vi "AlliGator Add Dataset to Accumulated Dataset.vi"(8 "error in (no error)":errorcluster, 9 "Weight (1)":dbl=1.0, 11 "AlliGator IV DVR in":refnum<data-value>) -> (0 "error out":errorcluster, 3 "AlliGator IV DVR out":refnum<data-value>)   [LabVIEW 2021, in "AlliGator Accumulated Dataset.lvlib"]
doc: "Adds the <B>Current Dataset</B> to the <B>Accumulated Dataset</B>, if and only if the number of gates and channels are the same as those of the first dataset in the series.\n\nIf not, the <B>Current Dataset</B> is skipped."
uses:
  AlliGator Accumulated Dataset.lvlib
  Internal Variables/AlliGator Internal Variables v2.ctl
  <vilib>/vision/Image Controls.llb/IMAQ Image.ctl
  Internal Variables/AlliGator Gate Image Set.ctl
  Files/AlliGator FLI Dataset Type.ctl
  Files/AlliGator Data Series Type.ctl
  Dual-Channel Datasets/AlliGator Dataset Channel.ctl
  Settings/AlliGator Gate Arithmetic.ctl
  Source Image/AlliGator Displayed Image.ctl
  Image/Named ROI Description.ctl
  Phasor Graph/AlliGator Decay Metadata v3.ctl
  Decay Analysis/Decay Preprocessing/AlliGator Decay Background Subtraction Info.ctl
  Decay Analysis/Decay Preprocessing/AlliGator Baseline Subtraction Method.ctl
  Graphs/XY Graph/XY Graph Plot Shift Parameters.ctl
  Graphs/XY Graph/XY Graph Plot Shift Method.ctl
  Decay Analysis/Decay Preprocessing/AlliGator Decay Extrapolation Parameters.ctl
  Phasor/Calibration Phasor (m, phi).ctl
  Phasor/Phasor Reference Series.ctl
  Phasor/Phasor Calibration Map v2.ctl
  Phasor/Phasor (g, s).ctl
  Phasor Graph/AlliGator Raw Phasor Plot Data v5.ctl
  Phasor/Phasor Standard Deviation Options.ctl
  Phasor Plot/AlliGator Phasor Multi-Harmonic Data.ctl
  Phasor/Phasor Harmonic Data.ctl
  Decay Fit Parameter Map/AlliGator Decay Fit Options & Parameters v4.ctl
  Fits/IRF(X)PSED/Decay Fit Options v4.ctl
  Fits/Decay Convolution/Decay Model.ctl
  Fits/Residual Type.ctl
  Fits/IRF(X)PSED/Fit Weights Type v2.ctl
  Fits/Non-linear Fitting Method v2.ctl
  Fits/Fit Calculation Method.ctl
  Fits/Non-linear Fitting Algorithm.ctl
  Decay Analysis/Decay Fit/AlliGator Decay Fit Parameter Constraints 2.ctl
  Fits/IRF(X)PSED/Decay Fit Parameters In List.ctl
  Fits/IRF(X)PSED/MLE Baseline Offset Type.ctl
  Decay Analysis/Decay Preprocessing/AlliGator Decay Preprocessing Parameters.ctl
  Fits/IRF(X)PSED/Decay Fit Parameters & Derived Quantities List v2.ctl
  Fits/IRF(X)PSED/Decay Fit Result Constraint.ctl
  Decay Fit Parameter Map/AlliGator Parameter Maps Data.ctl
  Globals, Variables, Constants/AlliGator Variables List.ctl
  Rich Text Box/Text Format List.ctl
  <vilib>/vision/NI_Vision_Development_Module.lvlib
  Globals, Variables, Constants/AlliGator Globals, Variables & Constants.lvlib
  Notebook/Notebook.lvlib
  Utilities/Utilities.lvlib
  Image/Image.lvlib
  Phasor/Phasor.lvlib
  Internal Variables/AlliGator Internal Variables.lvlib
  Files/AlliGator Files.lvlib
  Phasor Graph/AlliGator Phasor Graph.lvlib
  Decay Analysis/Decay Preprocessing/AlliGator Decay Preprocessing.lvlib
  Graphs/XY Graph/XY Graph Add-Ons.lvlib
  Phasor Plot/AlliGator Phasor Plot.lvlib
  Source Image/AlliGator Source Image.lvlib
  Fits/Fits.lvlib
  Decay Analysis/Decay Fit/AlliGator Decay Fit.lvlib
  Settings/AlliGator Settings.lvlib
  Dual-Channel Datasets/AlliGator Dual-Channel Datasets.lvlib
  Decay Fit Parameter Map/AlliGator Decay Fit Parameter Map.lvlib
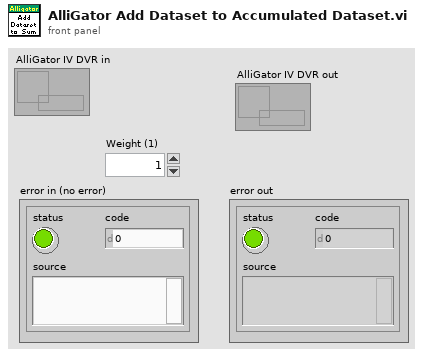
[diagram p1: front panel]
types:
  T1 = typedef "AlliGator Globals, Variables & Constants.lvlib/AlliGator Variables List.ctl" = enum16{"---- GUI ----", "GUI:Initialization Status", "GUI:State Indicators Refnum", "GUI:Original AlliGator Menu Items", "GUI:Current Action Loop State", "GUI:Script in progress", "GUI:Playback", "GUI:Loop Playback", "GUI:Search ROI Used", "GUI:Search ROI", "Decay Graph Max Legend Size", "Intensity Graph Max Legend Size", "Decay Statistics Graph Max Legend Size", "Phasor Graph Max Legend Size", "Phasor Ratio Graph Max Legend Size", "Lifetime Graph Max Legend Size", "---- Files ----", "Files:Export Dataset Frames as Individual Files", "Files:Show Batch Export Help Balloons", "Files:Frames in Dataset", "Files:ptu File Frame Start Indices", "Files:Current Frame in Dataset", "Files:Current Frame Timestamp", "Files:Dataset Loaded", "Files:Dataset Metadata", "Files:Dataset Channel", "Files:Dataset Data Description", "Files:Background Dataset Metadata", "Files:Background Dataset Channel", "Files:Background Dataset Data Description", "Files:Background File Subtraction", "Files:Background File Path", "Files:Background File Pile-up Correction", "Files:Background File Pixel Well Capacity", "Files:Background File Scaling Factor", "Files:Current Dataset Load Settings", "Files:Dataset Path", "Files:ICCD-specific Information", "Files:Macrotime Gate Separation", "------ Python Plugins ------", "Python Plugins:Information", "Python Plugins:Python Session", "Python Plugins:Valid Python Session?", "---- Source Image ----", "Source Image:ROIs", "Source Image:Current ROI", "Source Image:ROI Event Refnum", "X_Source Image:Display Range", "X_Source Image:Palette Information", "X_Source Image:Type of Displayed Image", "X_Time Gate Slider", "Source Image:Palette List", "Source Image:Scale", "Source Image:ROI Overlay Color", "Source Image:Overlay to Erase", "Source Image:Is Displayed Image Accumulated", "Source Image:White Light Image Modified", "Source Image:Mask Image Modified", "---- Image Profile Window ----", "Image Profile:Window Event Refnum", "Image Profile:IntensityType", "Image Profile:Intensity Average Type", "Image Profile:Intensity-weighted SDV", "Image Profile:Box Profile Type", "Image Profile:Window Open", "Image Profile:Plotted Fit Parameter", "------ Phasor Graph -------", "Phasor Graph:Show Line", "---- Phasor Plot ---", "Phasor Plot:Parameters Changed", "Phasor Plot:FLI Dataset Modified since last Calculation", "Phasor Harmonics Data", "Selected Phasor Harmonics", "Phasor Harmonic Manager Event Refnum", "Phasor Plot:ROIs", "Phasor Plot:Current ROI", "Phasor Plot:ROI Event Refnum", "Phasor Plot:Image Reference Points", "Phasor Plot:Computed", "Phasor Plot:Palette Information", "Phasor Plot:Palette List", "Phasor Plot:Phasor Ratio Palette Information", "Phasor Plot:Phasor Ratio Palette List", "Phasor Plot:Image Scale", "Phasor Plot:Image Overlay to Erase", "Phasor Plot:Image Elements to Update", "Phasor Plot:Current Calculation Parameters", "Phasor Plot:Current Calibration Options", "Phasor Plot:Reset Cumulated Phasor Plot", "Phasor Plot:Reference 1", "Phasor Plot:Lifetime Reference 1", "Phasor Plot:Reference 1 Frequency", "Phasor Plot:Reference 2", "Phasor Plot:Lifetime Reference 2", "Phasor Plot:Reference 2 Frequency", "---- Decay Analysis ----", "Number of Selected Decays to Fit", "LS Fit Results", "LAR Fit Results", "BS Fit Results", "Last Decay Max - Min", "Best Fit Parameters", "Best Fit Parameter Names", "Actual Size X", "Actual Size Y", "Binning X", "Binning Y", "Actual # Gates", "Dataset Number", "Gates to...", "Gates Skipped", "Gates to keep", "Gate Step", "Gate Separation", "Reversed Gates", "Pile-up Correction", "Pixel Well Capacity", "Background Subtracted", "Background Subtraction Method", "Background Definition Range", "Background File (deprecated)", "Number of Dataset Accumulated", "Array of Accumulated Dataset Paths", "Do Averaged Datasets", "Destination File Path", "Process Plot Target", "Use 1/D as Phasor Frequency", "---- Decay Fit Parameter Map -----", "Decay Fit Parameter Map:Palette Information", "Decay Fit Parameter Map:Palette List", "Decay Fit Parameter Map:X Resolution", "Decay Fit Parameter Map:Y Resolution", "Decay Fit Parameter Map:Use Decay Fit Result Constraints", "Decay Fit Parameter Map:Decay Fit Result Constraints", "Decay Fit Parameter Map:Decay Fit Result Constraints Applied", "---- Parameter Map ----", "Parameter Map:Palette Information", "Parameter Map:Palette List", "------- Local Decay Window ---------", "Local Decay Graph Window:Event Refnum", "Local Decay Graph Window:Use normalized IRF for convolution", "----- Miscellaneous ----", "Misc:Skippable Dialog Windows Status"}
  T2 = enum32{"Average", "Min", "Max", "Clear  if < ", "Clear  if < or =", "Clear  if =", "Clear  if > or =", "Clear  if >"}
  T3 = typedef "Notebook.lvlib/Text Format List.ctl" = enum16{"Message", "Result", "Error", "Setting", "Verbose", "Warning"}
  T4 = typedef "AlliGator Internal Variables.lvlib/AlliGator Internal Variables v2.ctl" = cluster{"----------------------------- Images -----------------------------":u8, "Displayed Image":T5, "White Light Image":T5, "Mask Image":T5, "ROI Mask Image":T5, "Current Dataset Images 1":T6, "Background Dataset Images 1":T6, "Current Dataset Images 2":T6, "Background Dataset Images 2":T6, "Current Dataset Arithmetic Images":T6, "Accumulated Dataset Images 1":T6, "Accumulated Dataset Images 2":T6, "Accumulated Dataset Arithmetic Images":T6, "----------------------------- File Paths -----------------------------":u8, "Phasor Plot Image":T5, "Decay Fit Parameter Map Image":T5, "Parameter Map Image":T5, "Single Data Point Path":path, "White Light Image Path":path, "Mask Image Path":path, "Time-Series Folder":path, "[Time-Series Paths]":path[], "----------------------------- FLI Dataset -----------------------------":u8, "Current Dataset":i32, "Single Dataset Type":T7, "Current Folder":string, "AlliGator Data Series Type":T8, "# Datasets":i32, "Dual-Channel Dataset":bool, "Selected Channel Name":string, "Dataset Channel":T9, "Channel Arithmetic":T10, "Dual-Channel Background Dataset":bool, "Background Channel":T9, "Dual-Channel Accumulated Dataset":bool, "Start Time":dbl, "[Time-Series Timestamps]":dbl[], "[Intensity Corrections]":dbl[], "Time Series Script":bool, "Type of Displayed Image":T11, "Gate Image Slide":u16, "# Gates":i32, "ROIs":T12[], "----------------------------- Decays -----------------------------":u8, "ROI Decay":cluster{"t Array":dbl[], "I Array":dbl[]}, "Valid Decay":bool, "Decay  Metadata":T14, "Reference Decay Plot Name":string, "Reference Decay":cluster{"t Array":dbl[], "I Array":dbl[]}, "Decay Shift Plot":cluster{"Time Stamps":dbl[], "Decay Shifts":dbl[]}, "[Decays Max Values]":sgl[], "[Decays Min Values]":sgl[], "----------------------------- Calibration -----------------------------":u8, "Calibration Phasor":T20, "Calibration Phasor Series":T21, "Phasor Calibration Map":T22, "Calibration Map MD5 Digest":string, "----------------------------- Phasor Graph -----------------------------":u8, "Last Raw Phasor":T23, "Last Calibrated Phasor":T23, "Last Calibrated Phasor SDV":T23, "Phasor Graph:Phasor Plot":cluster{"g Array":dbl[], "s Array":dbl[]}, "Phasor Graph:Phasor SDV Plot":cluster{"g Array":dbl[], "s Array":dbl[]}, "[Phasor Graph:Raw Phasor Plots]":T24[], "Phasor Plot locked to Ref 1":i32, "[Phasor Plot(s) locked to Ref 1]":i32[], "[Phasor Plot(s) locked to Ref 2]":i32[], "[Pixel Phasors]":T23[], "----------------------------- Phasor Plot -----------------------------":u8, "[[Sum Image]]":dbl[][], "[[CSG Phasors]]":csg[][], "[[Valid Pixel?]]":bool[][], "[[Phasor Ratios]]":dbl[][], "[[Average Lifetimes]]":dbl[][], "Amplitude Weighted Average Lifetime":bool, "I/m/phi Dataset":cluster{"I/m/phi Dataset?":bool, "Base Frequency":dbl[unit], "Harmonic Orders":u8[]}, "Multi Phasor Plot Data":T26, "----------------------------- Decay Fit Parameter Map -----------------------------":u8, "Decay Fit Options & Parameters":T28, "Fit Options: Decay Preprocessing Parameters":T39, "Fit Options: Reference Decay":cluster{"t Array":dbl[], "I Array":dbl[]}, "Is Full Image Parameters Map":bool, "Is Single-Pixels Parameters Map":bool, "NLSF Parameters Map X Resolution":i32, "NLSF Parameters Map Y Resolution":i32, "[Single Decay Fit Parameters]":dbl[], "Fit Model":T30, "[[Multiple Decays Fit Parameters]]":dbl[][], "[[Multiple Decays Fit Parameter SDVs]]":dbl[][], "[[IRFs]]":dbl[][], "[ROI Descriptors]":T13[], "IRF Array Time Axis":dbl[], "Decay Array Time Axis":dbl[], "[Decay Fit Parameter Names]":T40[], "[Decay Sum]":dbl[], "Array of Decay Fit Result Constraints":T41[], "Selected ROIs Array":bool[], "----------------------------- Parameter Maps -----------------------------":u8, "[Map Set Names]":string[], "[Parameter Maps]":T42[], "[[User-defined Quantities]]":dbl[][], "User-defined Quantity":string}
  T5 = typedef "IMAQ Image.ctl" = refnum<image>
  T6 = typedef "AlliGator Internal Variables.lvlib/AlliGator Gate Image Set.ctl" = cluster{"SGL Gate Images":T5[], "SGL Sum Image":T5, "SGL Max Image":T5, "SGL Min Image":T5}
  T7 = typedef "AlliGator Files.lvlib/AlliGator FLI Dataset Type.ctl" = enum16{"HDF5 FLI Dataset", "Gate Image Folder", ".sdt FLI Dataset (Becker & Hickl)", ".ptu FLI Dataset (PicoQuant)", "SS1 FLI Dataset", "SS2 FLI Dataset", "I/m/phi Dataset", ".bin FLI Dataset (PicoQuant Binned)", ".bin FLI Dataset (Piccolo Binned)", ".mat FLI Dataset"}
  T8 = typedef "AlliGator Files.lvlib/AlliGator Data Series Type.ctl" = enum16{"Not a Supported Series", "Gate Images Folder Series", "SwissSPAD 2 Dataset Series", "B&H FLI Dataset Series", "PicoQuant PTU FLI Dataset Series", "PicoQuant BIN FLI Dataset Series", "Piccolo hist BIN FLI Dataset Series", "HDF5 FLI Dataset Series"}
  T9 = typedef "AlliGator Dual-Channel Datasets.lvlib/AlliGator Dataset Channel.ctl" = enum16{"G2", "INT"}
  T10 = typedef "AlliGator Settings.lvlib/AlliGator Gate Arithmetic.ctl" = enum16{"None", "INT-G2", "G2/INT*<INT>", "(1 - G2/INT)*<INT>"}
  T11 = typedef "AlliGator Source Image.lvlib/AlliGator Displayed Image.ctl" = enum16{"Single Gate", "Sum of All Gates", "Max of All Gates", "Min of All Gates", "-", "White Ligth Image", "Mask Image"}
  T12 = typedef "Image.lvlib/Named ROI Description.ctl" = cluster{"ROI Descriptor":T13, "ROI Name":string, "Overlay Color":u32}
  T13 = typedef "ROI Descriptor" = cluster{"Global Rectangle":i32[], "Contours":cluster{"ID":enum32{"External", "Internal"}, "Type":u32, "Coordinates":i32[]}[]}
  T14 = typedef "AlliGator Phasor Graph.lvlib/AlliGator Decay Metadata v3.ctl" = cluster{"ROI Descriptor":T13, "ROI Center":cluster{"X":i32, "Y":i32}, "Decay Background Subtraction Info":T15, "Decay Reverted":bool, "Decay Smoothened":bool, "Decay Straightened":bool, "Fitted Tau (Decay Straightening)":dbl, "Decay Shift Parameters":T17, "Decay Shifted":bool, "Decay Extrapolated":bool, "Decay Extrapolation Parameters":T19, "Decay Normalized":bool, "Fold Decay":bool, "# Folds":u32}
  T15 = typedef "AlliGator Decay Preprocessing.lvlib/AlliGator Decay Background Subtraction Info.ctl" = cluster{"Laser Period":dbl[unit], "Gate Duration":dbl[unit], "Baseline Subtraction Method":T16, "Background Definition Range":cluster{"Min Gate":dbl[unit], "Max Gate":dbl[unit]}, "Total Intensity w/o Bkgd Subtraction":dbl, "Bkgd-subtracted Intensity (exp)":dbl, "# Data Points":i32, "Background/Gate":dbl, "Fitted Lifetime":dbl[unit], "Bkgd-subtracted Intensity (theo)":dbl}
  T16 = typedef "AlliGator Decay Preprocessing.lvlib/AlliGator Baseline Subtraction Method.ctl" = enum16{"Mean", "Min", "Square Gated Single-Exponential", "File", "Constant"}
  T17 = typedef "XY Graph Add-Ons.lvlib/XY Graph Plot Shift Parameters.ctl" = cluster{"Type":T18, "Shift":dbl[unit], "Threshold":dbl, "Rotate":bool}
  T18 = typedef "XY Graph Add-Ons.lvlib/XY Graph Plot Shift Method.ctl" = enum16{"Default", "CFD", "Threshold", "Cross-Correlation"}
  T19 = typedef "AlliGator Decay Preprocessing.lvlib/AlliGator Decay Extrapolation Parameters.ctl" = cluster{"Additional Points":u32, "Head Fraction":dbl, "Fitted Tau":dbl, "Use Periodicity":bool, "Use Cursors":bool, "Tail Fraction":dbl}
  T20 = typedef "Phasor.lvlib/Calibration Phasor (m, phi).ctl" = cluster{"m":dbl, "phi":dbl, "Phasor Frequency":dbl[unit], "Reference Lifetime":dbl[unit]}
  T21 = typedef "Phasor.lvlib/Phasor Reference Series.ctl" = cluster{"m Array":dbl[], "phi Array":dbl[], "Phasor Frequency":dbl[unit], "Calibration Lifetime":dbl[unit]}
  T22 = typedef "Phasor.lvlib/Phasor Calibration Map v2.ctl" = cluster{"Phasor Frequency":dbl[unit], "Calibration Lifetime":dbl[unit], "ROI Centers":cluster{"X":i32, "Y":i32}[], "ROI Descriptors":T13[], "Map Resolution X":i32, "Map Resolution Y":i32, "z Array":cdb[]}
  T23 = typedef "Phasor.lvlib/Phasor (g, s).ctl" = cluster{"g":dbl, "s":dbl}
  T24 = typedef "AlliGator Phasor Graph.lvlib/AlliGator Raw Phasor Plot Data v5.ctl" = cluster{"Phasor Plot Name":string, "Raw Phasor Plot":T23[], "Phasor Frequency":dbl[unit], "[Decay Metadata]":T14[], "Raw Phasor Plot SDV":T23[], "Phasor SDV Options":T25, "[Calibration Phasor]":T20[], "Intensity Array":dbl[]}
  T25 = typedef "Phasor.lvlib/Phasor Standard Deviation Options.ctl" = cluster{"Compute Estimated SDV":bool, "# Replicas":u32, "Use Estimated Average Phasor":bool}
  T26 = typedef "AlliGator Phasor Plot.lvlib/AlliGator Phasor Multi-Harmonic Data.ctl" = cluster{"Base Frequency":dbl[unit], "# Harmonics":u8, "Harmonic Orders":u8[], "Phasor Plot Settings Checksum":u64, "Phasor Harmonic Data Array":T27[]}
  T27 = typedef "Phasor.lvlib/Phasor Harmonic Data.ctl" = cluster{"Phasor Harmonic Name":string, "Phasor Plot Settings Checksum":u64, "Phasor Frequency":dbl[unit], "Base Frequency":dbl[unit], "Harmonic Order":u8, "Phasor Plot Parameters":string, "Phasor Array [[CSG]]":csg[][], "Dataset File Path":path}
  T28 = typedef "AlliGator Decay Fit Parameter Map.lvlib/AlliGator Decay Fit Options & Parameters v4.ctl" = cluster{"SYNC Period":dbl[unit], "Fit Options":T29, "Fit Parameter Constraints":T36[], "MLE Baseline Offset":dbl, "MLE Baseline Offset Type":T38}
  T29 = typedef "Fits.lvlib/Decay Fit Options v4.ctl" = cluster{"Show Fit Residuals":bool, "Fit Model":T30, "Residual Type":T31, "Max Decay Percentile":dbl, "Min Decay Percentile":dbl, "Show Full Decay":bool, "Weights":T32, "Fitting Method":T33, "Compute Parameter Uncertainties":bool, "Periodic Boundaries":bool, "Model Calculation":T34, "Period":dbl[unit], "Termination Criteria":cluster{"Max Iterations":i32, "Max Function Calls":i32, "Max Time":dbl[unit], "Function Tolerance":dbl, "Parameter Tolerance":dbl, "Gradient Tolerance":dbl, "Min Lambda":dbl, "Max Lambda":dbl, "Initial Tick Count":u32}, "Offset Resolution":dbl[unit], "Use Local IRF":bool, "Fitting Algorithm":T35, "Show Confidence Interval ":bool, "Confidence Level":dbl}
  T30 = typedef "Fits.lvlib/Decay Model.ctl" = enum16{"1-Exponential", "2-Exponentials"}
  T31 = typedef "Fits.lvlib/Residual Type.ctl" = enum16{"Standard", "Normalized", "Reduced"}
  T32 = typedef "Fits.lvlib/Fit Weights Type v2.ctl" = enum16{"Unweighted", "1/Variance (Neyman)", "1/Variance (Pearson)", "Best of All"}
  T33 = typedef "Fits.lvlib/Non-linear Fitting Method v2.ctl" = enum16{"Least Square", "Least Absolute Residual", "Bisquare", "MLE", "-", "Best of All"}
  T34 = typedef "Fits.lvlib/Fit Calculation Method.ctl" = enum16{"Simulation", "Convolution", "Integration"}
  T35 = typedef "Fits.lvlib/Non-linear Fitting Algorithm.ctl" = enum16{"Levenberg-Marquardt", "Trust-Region Dogleg"}
  T36 = typedef "AlliGator Decay Fit.lvlib/AlliGator Decay Fit Parameter Constraints 2.ctl" = cluster{"Fit Parameter":T37, "Min Value":dbl, "Max Value":dbl, "Global":bool, "Used":bool}
  T37 = typedef "Fits.lvlib/Decay Fit Parameters In List.ctl" = enum16{"Offset", "Baseline", "A_1", "tau_1", "A_2", "tau_2"}
  T38 = typedef "Fits.lvlib/MLE Baseline Offset Type.ctl" = enum32{"Absolute", "Percentage"}
  T39 = typedef "AlliGator Decay Preprocessing.lvlib/AlliGator Decay Preprocessing Parameters.ctl" = cluster{"Background Subtraction":bool, "Straighten Decay":bool, "Reverse Gates":bool, "1-Normalized Decay":bool, "Smoothen Decay":bool, "Smoothing Parameter":dbl, "Shift Decay":bool, "Decay Shift Parameters":T17, "Extrapolate Decay":bool, "Additional Points":u32, "Head Fraction":dbl, "Pixel-Normalize Decay":bool, "Use Periodicity":bool, "Use Cursors":bool, "Tail Fraction":dbl, "Use Decay Pre-Processing":bool, "Fold Decay":bool, "# Folds":u32, "[0-1]-Normalized Decay":bool}
  T40 = typedef "Fits.lvlib/Decay Fit Parameters & Derived Quantities List v2.ctl" = enum16{"Offset", "Baseline", "A_1", "tau_1", "A_2", "tau_2", "<tau>_a", "f1_a", "f2_a", "<tau>_i", "f1_i", "f2_i", "-", "R^2", "Chi^2"}
  T41 = typedef "Fits.lvlib/Decay Fit Result Constraint.ctl" = cluster{"Fit Parameter":enum16{"Offset", "Baseline", "A_1", "tau_1", "A_2", "tau_2", "<tau>_a", "f1_a", "f2_a", "<tau>_i", "f1_i", "f2_i", "-", "R^2", "Chi^2", "Max Relative Residual", "<Residual ACF>", "Residual ACF SDV", "tau_2/tau_1"}, "Min Value":dbl, "Max Value":dbl, "Use Constraint":bool}
  T42 = typedef "AlliGator Decay Fit Parameter Map.lvlib/AlliGator Parameter Maps Data.ctl" = cluster{"Map Set Name":string, "[Parameter Names]":string[], "[[Parameters]]":dbl[][], "[[Parameter SDVs]]":dbl[][], "Decay Array Time Axis":dbl[], "[[IRFs]]":dbl[][], "IRF Array Time Axis":dbl[], "X Resolution":i32, "Y Resolution":i32, "Intensity Array":dbl[]}
  T43 = typedef "Rich Text Box.lvlib/Text Formatting.ctl" = cluster{"Font":string, "Text Color":T44, "Background Color":T44, "Style":T45, "Font Size":dbl, "Alignment":T46}
  T44 = typedef "Rich Text Box.lvlib/Text Colors.ctl" = enum16{"Unchanged", "Black", "Blue", "Cyan", "Maroon", "Gray", "Violet", "Green", "Light Green", "Orange", "Yellow", "Magenta", "Red", "White"}
  T45 = typedef "Rich Text Box.lvlib/Text Style.ctl" = enum16{"Regular", "Bold", "Italic", "Underline", "Strikeout"}
  T46 = typedef "Rich Text Box.lvlib/Text Alignment.ctl" = enum16{"Left", "Right", "Center"}
  T47 = typedef "Image Type" = u32
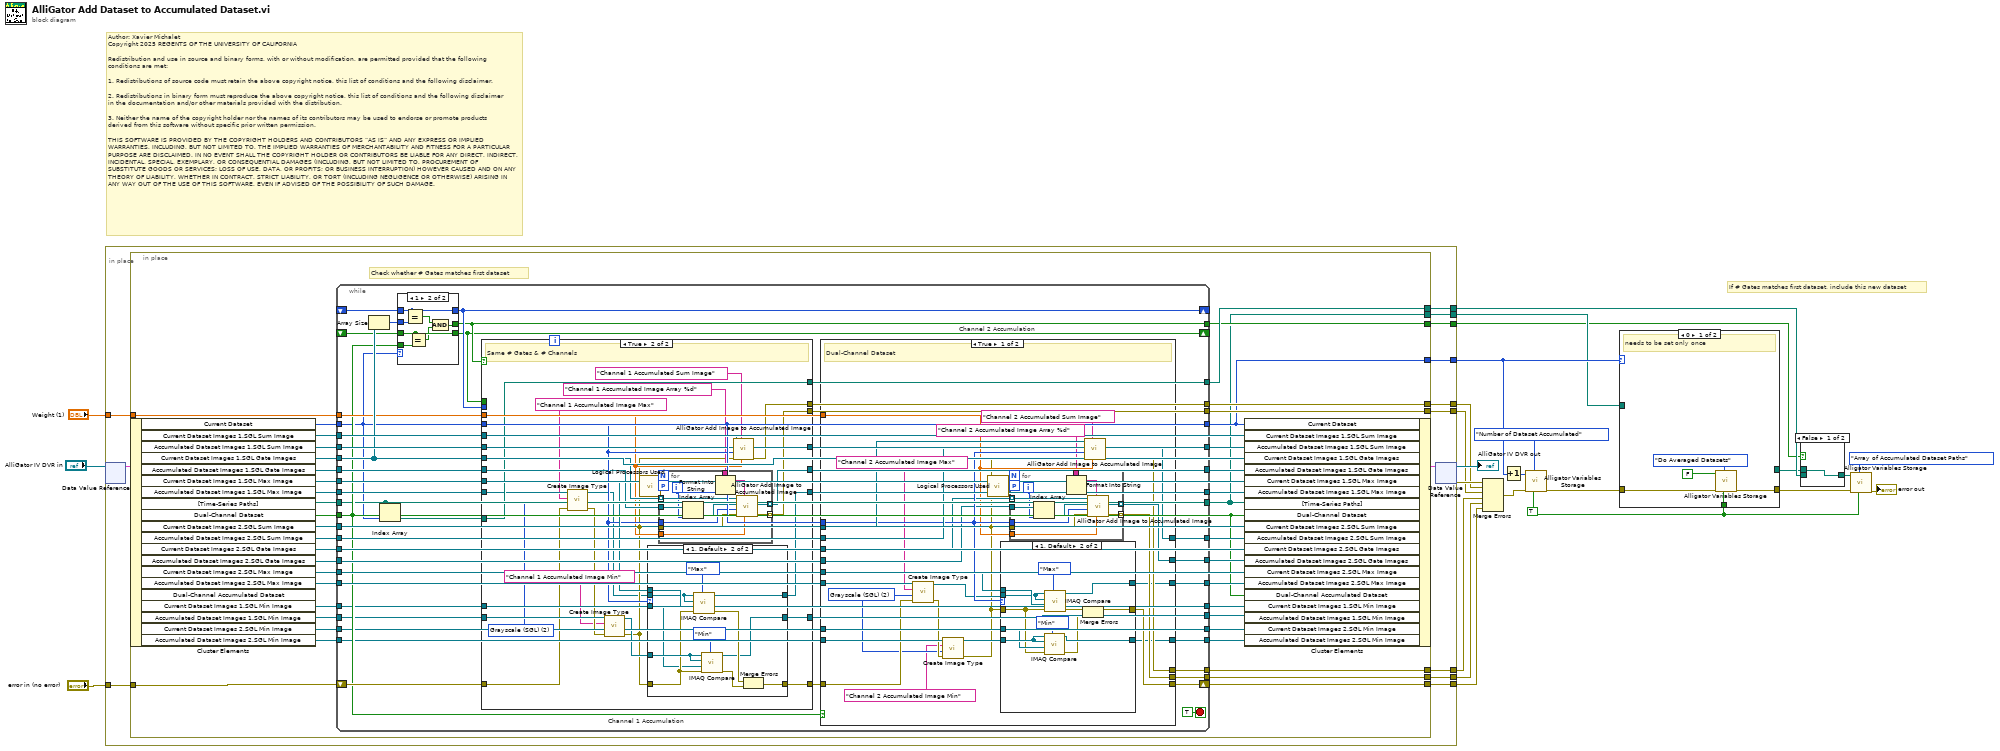
[diagram p0: block diagram]
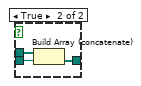
[diagram p2: hidden frame]
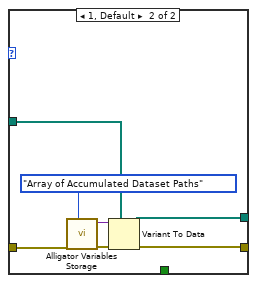
[diagram p3: hidden frame]
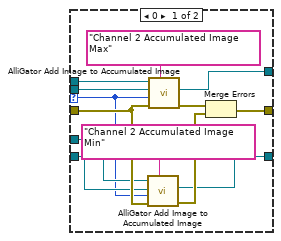
[diagram p4: hidden frame]
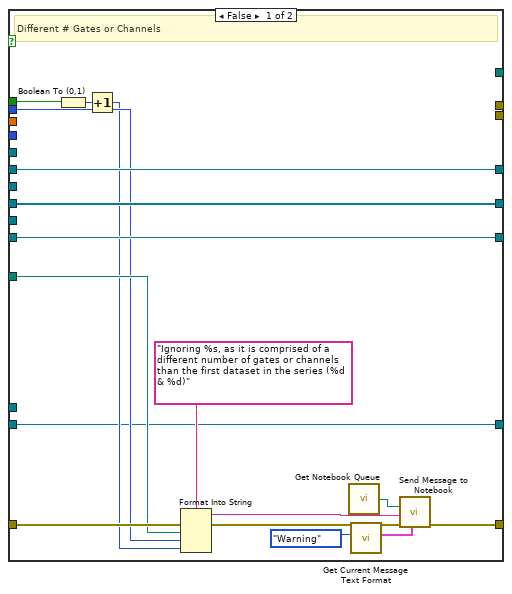
[diagram p6: hidden frame]
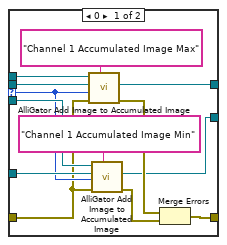
[diagram p7: hidden frame]
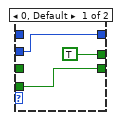
[diagram p8: hidden frame]
diagram:
  w5 = TRUE ("Get(F)/Set")
  # "Author: Xavier Michalet\nCopyright 2025 REGENTS OF THE UNIVERSITY OF CALIFORNIA\n\nRedistribution and use in source and binary forms, with or without modification, are permitted provided that the following conditions are met:\n\n1. Redistributions of source code must retain the above copyright notice, this list of conditions and the following disclaimer.\n\n2. Redistributions in binary form must reproduce the above copyright notice, this list of conditions and the following disclaimer in the documentation and/or other materials provided with the distribution.\n\n3. Neither the name of the copyright holder nor the names of its contributors may be used to endorse or promote products derived from this software without specific prior written permission.\n\nTHIS SOFTWARE IS PROVIDED BY THE COPYRIGHT HOLDERS AND CONTRIBUTORS “AS IS” AND ANY EXPRESS OR IMPLIED WARRANTIES, INCLUDING, BUT NOT LIMITED TO, THE IMPLIED WARRANTIES OF MERCHANTABILITY AND FITNESS FOR A PARTICULAR PURPOSE ARE DISCLAIMED. IN NO EVENT SHALL THE COPYRIGHT HOLDER OR CONTRIBUTORS BE LIABLE FOR ANY DIRECT, INDIRECT, INCIDENTAL, SPECIAL, EXEMPLARY, OR CONSEQUENTIAL DAMAGES (INCLUDING, BUT NOT LIMITED TO, PROCUREMENT OF SUBSTITUTE GOODS OR SERVICES; LOSS OF USE, DATA, OR PROFITS; OR BUSINESS INTERRUPTION) HOWEVER CAUSED AND ON ANY THEORY OF LIABILITY, WHETHER IN CONTRACT, STRICT LIABILITY, OR TORT (INCLUDING NEGLIGENCE OR OTHERWISE) ARISING IN ANY WAY OUT OF THE USE OF THIS SOFTWARE, EVEN IF ADVISED OF THE POSSIBILITY OF SUCH DAMAGE."
  # "If # Gates matches first dataset, include this new dataset"
  n1 = in-place {
    in-place-border: "error in (no error)" -> [w35]
    in-place-border: [w34] -> w20
    in-place-border: [w33] -> w19
    in-place-border: [w32] -> w18
    in-place-border: [w31] -> w12
    in-place-border: [w30] -> w15
    in-place-border: [w29] -> w10
    in-place-border: [w28] -> w4
    in-place-border: "Weight (1)" -> [w27]
    in-place-border: [w26] -> w2
    in-place-border: [w25] -> w1
    n2 = in-place-dvr #1("AlliGator IV DVR in") -> (w37:T4)  [unwired: 1 out]
    n3 = in-place {
      in-place-border: w35 -> [w67]
      in-place-border: [w71] -> w34
      in-place-border: [w70] -> w33
      in-place-border: [w66] -> w32
      in-place-border: [w61] -> w31
      in-place-border: [w64] -> w30
      in-place-border: [w47] -> w29
      in-place-border: [w60] -> w28
      in-place-border: w27 -> [w59]
      in-place-border: [w49] -> w26
      in-place-border: [w48] -> w25
      # "Check whether # Gates matches first dataset"
      n4 = in-place-cluster #2(w37) -> ("Current Dataset"=w62:i32, "Current Dataset Images 1.SGL Sum Image"=w75:T5, "Accumulated Dataset Images 1.SGL Sum Image"=w77:T5, "Current Dataset Images 1.SGL Gate Images"=w72:T5[], "Accumulated Dataset Images 1.SGL Gate Images"=w74:T5[], "Current Dataset Images 1.SGL Max Image"=w68:T5, "Accumulated Dataset Images 1.SGL Max Image"=w69:T5, "[Time-Series Paths]"=w63:path[], "Dual-Channel Dataset"=w46:bool, "Current Dataset Images 2.SGL Sum Image"=w56:T5, "Accumulated Dataset Images 2.SGL Sum Image"=w58:T5, "Current Dataset Images 2.SGL Gate Images"=w55:T5[], "Accumulated Dataset Images 2.SGL Gate Images"=w54:T5[], "Current Dataset Images 2.SGL Max Image"=w53:T5, "Accumulated Dataset Images 2.SGL Max Image"=w52:T5, "Current Dataset Images 1.SGL Min Image"=w45:T5, "Accumulated Dataset Images 1.SGL Min Image"=w44:T5, "Current Dataset Images 2.SGL Min Image"=w41:T5, "Accumulated Dataset Images 2.SGL Min Image"=w39:T5)  [unwired: 1 out]
      n5 = while {
        tunnel: w75 -> [w119]
        tunnel: w72 -> [w110]
        tunnel: [w117] -> w71
        tunnel: [w116] -> w70
        tunnel: w68 -> [w114]
        tunnel: [w104] -> w64
        tunnel: w63 -> [w85]
        tunnel: w62 -> [w84]
        shift-right: [w101] -> w66
        shift-left: w67 -> [w113]
        tunnel: w77 -> [w121]
        tunnel: [w120] -> w76
        tunnel: w74 -> [w111]
        tunnel: [w118] -> w73
        tunnel: w69 -> [w115]
        tunnel: [w112] -> w65
        shift-right: [w106] -> _
        shift-left: _ -> [w109]
        tunnel: [w84] -> w61
        tunnel: [w103] -> w60
        tunnel: w59 -> [w93]
        tunnel: w56 -> [w100]
        tunnel: w58 -> [w99]
        tunnel: [w98] -> w57
        tunnel: w55 -> [w97]
        tunnel: w54 -> [w96]
        tunnel: w53 -> [w95]
        tunnel: w52 -> [w94]
        tunnel: [w92] -> w51
        tunnel: [w91] -> w50
        tunnel: [w90] -> w49
        tunnel: [w89] -> w48
        tunnel: w46 -> [w88]
        shift-right: [w86] -> _
        shift-left: _ -> [w87]
        tunnel: [w85] -> w47
        tunnel: w45 -> [w81]
        tunnel: w44 -> [w83]
        tunnel: [w82] -> w42
        tunnel: [w81] -> w43
        tunnel: w41 -> [w78]
        tunnel: [w78] -> w40
        tunnel: w39 -> [w80]
        tunnel: [w79] -> w38
        stop <- TRUE stop-if-true
        n6 = Array Size(array=w110) -> (size(s)=w105:i32)
        n7 = Index Array(array=w85, index=w84) -> (element=w107:path)
        n8 = case shown="1" w84 {
          tunnel: w105 -> [w275 w282]
          tunnel: [w275 w281] -> w106
          tunnel: w109 -> [_ w281]
          tunnel: [TRUE w277] -> w103
          tunnel: w88 -> [w273 w279]
          tunnel: [w273 w278] -> w86
          tunnel: w87 -> [_ w278]
          frame 0, Default {
          }
          frame 1 {
            n9 = Equal?(x=w281, y=w282) -> (x = y?=w280:bool)
            n10 = Equal?(x=w278, y=w279) -> (x = y?=w276:bool)
            n11 = Compound Arithmetic op=AND(w280, w276) -> (w277:bool)
          }
        }
        n12 = case "Channel 1 Accumulation" shown="True" w103 {
          tunnel: w121 -> [w207 w236]
          tunnel: [w207 w235] -> w120
          tunnel: w119 -> [_ w234]
          tunnel: [w206 w233] -> w118
          tunnel: [_ w232] -> w117
          tunnel: [_ w231] -> w116
          tunnel: w115 -> [w205 w219]
          tunnel: w114 -> [_ w230]
          tunnel: w113 -> [w199 w209]
          tunnel: [w200 w229] -> w102
          tunnel: [w205 w228] -> w112
          tunnel: w84 -> [_ w227]
          tunnel: w111 -> [w206 w226]
          tunnel: w110 -> [_ w225]
          tunnel: w107 -> [w198 w222]
          tunnel: w106 -> [w196 _]
          tunnel: [_ w222] -> w104
          tunnel: w93 -> [_ w224]
          tunnel: w86 -> [w195 _]
          tunnel: w81 -> [_ w221]
          tunnel: w83 -> [w192 w215]
          tunnel: [w192 w220] -> w82
          frame False {
            # "Different # Gates or Channels"
            n13 = Boolean To (0,1)(Boolean=w195) -> (0, 1=w194:i16)
            n14 = Increment(x=w194) -> (x+1=w193:i16)
            n15 = Format Into String(format string="Ignoring %s, as it is comprised of a different number of gates or channels  than the first dataset in the series (%d & %d)", error in=w199, w198, w196, w193) -> (resulting string=w202:string, error out=w201:errorcluster)  [unwired: 1 in]
            n16 = call "Get Notebook Queue.vi"() -> ("Notebook Queue"=w204:refnum<queue>)  [unwired: 9 in]
            n17 = call "Get Current Message Text Format.vi"("Text Format"=Text_Format_List."Warning") -> ("Message Formatting"=w203:T43)  [unwired: 8 in, 1 out]
            n18 = call "Send Message to Notebook.vi"("Text Formatting"=w203, "Error In"=w201, "Text"=w202, "Notebook Queue"=w204) -> ("Error Out"=w200:errorcluster)  [unwired: 4 in, 1 out]
          }
          frame True {
            w212 = T47 2 items=["Grayscale (U8)", "Grayscale (I16)", "Grayscale (SGL)", "Complex (CSG)", "RGB (U32)", "HSL (U32)", "RGB (U64)", "Grayscale (U16)"] ("Image Type")
            # "Same # Gates & # Channels"
            n19 = call "Create Image Type.vi"("error in (no error)"=w209, "Image Type"=w212, "Image Name"="Channel 1 Accumulated Image Max", "Refnum in"=w219) -> ("error out"=w213:errorcluster, "Refnum out"=w208:T5)  [unwired: 5 in, 1 out]
            n20 = call "Create Image Type.vi"("error in (no error)"=w213, "Image Type"=w212, "Image Name"="Channel 1 Accumulated Image Min", "Refnum in"=w215) -> ("error out"=w210:errorcluster, "Refnum out"=w214:T5)  [unwired: 5 in, 1 out]
            n21 = call "Logical Processors Used.vi"() -> ("# Logical Processor Used"=w223:i32)  [unwired: 6 in]
            n22 = case shown="1, Default" w227 {
              selector: w227 -> [w241 _]
              tunnel: w208 -> [w248 w257]
              tunnel: w230 -> [w249 w260]
              tunnel: w210 -> [w240 w255]
              tunnel: [w239 w251] -> w229
              tunnel: [w246 w258] -> w228
              tunnel: w221 -> [w243 w254]
              tunnel: w214 -> [w242 w256]
              tunnel: [w237 w252] -> w220
              frame 0 {
                n23 = call "AlliGator Add Image to Accumulated Image.vi"("Image Name"="Channel 1 Accumulated Image Max", "Error In"=w240, "Dataset Index"=w241, "Accumulated Image Sum (in("=w248, "New Image"=w249) -> ("Error Out"=w247:errorcluster, "Accumulated Image Sum (out)"=w246:T5)  [unwired: 5 in]
                n24 = call "AlliGator Add Image to Accumulated Image.vi"("Image Name"="Channel 1 Accumulated Image Min", "Error In"=w240, "Dataset Index"=w241, "Accumulated Image Sum (in("=w242, "New Image"=w243) -> ("Error Out"=w238:errorcluster, "Accumulated Image Sum (out)"=w237:T5)  [unwired: 5 in]
                n25 = Merge Errors(w247, w238) -> (w239:errorcluster)
              }
              frame 1, Default {
                n26 = call "IMAQ Compare"("Operator"=T2."Max", "error in (no error)"=w255, "Image Src B"=w260, "Image Dst"=w257, "Image Src A"=w257) -> ("error out"=w259:errorcluster, "Image Dst Out"=w258:T5)  [unwired: 5 in]
                n27 = call "IMAQ Compare"("Operator"=T2."Min", "error in (no error)"=w255, "Image Src B"=w254, "Image Dst"=w256, "Image Src A"=w256) -> ("error out"=w250:errorcluster, "Image Dst Out"=w252:T5)  [unwired: 5 in]
                n28 = Merge Errors(w259, w250) -> (w251:errorcluster)
              }
            }
            n29 = for {
              tunnel: w225 -> [w272] mode=indexing
              tunnel: w226 -> [w271]
              tunnel: [w270] -> w232 mode=indexing
              tunnel: w210 -> [w269]
              tunnel: w227 -> [w268]
              tunnel: "Channel 1 Accumulated Image Array %d" ("Image Name") -> [w267]
              tunnel: [w263] -> w233 mode=indexing
              workers-P: w223 -> [_]
              tunnel: w224 -> [w262]
              i -> [w264]
              n30 = Index Array(array=w271, index=w264) -> (element=w265:T5)
              n31 = Format Into String(format string=w267, w264) -> (resulting string=w266:string)  [unwired: 2 in, 1 out]
              n32 = call "AlliGator Add Image to Accumulated Image.vi"("Weight (1)"=w262, "Image Name"=w266, "Error In"=w269, "Dataset Index"=w268, "Accumulated Image Sum (in("=w265, "New Image"=w272) -> ("Error Out"=w270:errorcluster, "Accumulated Image Sum (out)"=w263:T5)  [unwired: 4 in]
            }
            n33 = call "AlliGator Add Image to Accumulated Image.vi"("Weight (1)"=w224, "Image Name"="Channel 1 Accumulated Sum Image", "Error In"=w210, "Dataset Index"=w227, "Accumulated Image Sum (in("=w236, "New Image"=w234) -> ("Error Out"=w231:errorcluster, "Accumulated Image Sum (out)"=w235:T5)  [unwired: 4 in]
          }
        }
        n34 = case "Channel 2 Accumulation" shown="True" w88 {
          tunnel: w99 -> [w149 w190]
          tunnel: w100 -> [w148 _]
          tunnel: [w147 w189] -> w92
          tunnel: [w146 _] -> w89
          tunnel: [w145 _] -> w90
          tunnel: w102 -> [w125 w187]
          tunnel: [w144 w187] -> w101
          tunnel: [w143 w188] -> w98
          tunnel: w84 -> [w142 _]
          tunnel: w97 -> [w140 _]
          tunnel: w96 -> [w139 w189]
          tunnel: w95 -> [w138 _]
          tunnel: w94 -> [w131 w188]
          tunnel: w93 -> [w137 _]
          tunnel: [w136 w190] -> w91
          tunnel: w80 -> [w129 w186]
          tunnel: [w134 w186] -> w79
          tunnel: w78 -> [w135 _]
          frame True {
            w124 = T47 2 items=["Grayscale (U8)", "Grayscale (I16)", "Grayscale (SGL)", "Complex (CSG)", "RGB (U32)", "HSL (U32)", "RGB (U64)", "Grayscale (U16)"] ("Image Type")
            # "Dual-Channel Dataset"
            n35 = call "Create Image Type.vi"("error in (no error)"=w125, "Image Type"=w124, "Image Name"="Channel 2 Accumulated Image Max", "Refnum in"=w131) -> ("error out"=w127:errorcluster, "Refnum out"=w130:T5)  [unwired: 5 in, 1 out]
            n36 = call "Create Image Type.vi"("error in (no error)"=w127, "Image Type"=w124, "Image Name"="Channel 2 Accumulated Image Min", "Refnum in"=w129) -> ("error out"=w126:errorcluster, "Refnum out"=w128:T5)  [unwired: 5 in, 1 out]
            n37 = call "Logical Processors Used.vi"() -> ("# Logical Processor Used"=w141:i32)  [unwired: 6 in]
            n38 = case shown="1, Default" w142 {
              selector: w142 -> [w150 _]
              tunnel: w130 -> [w161 w170]
              tunnel: w138 -> [w162 w173]
              tunnel: w126 -> [w156 w167]
              tunnel: [w155 w165] -> w144
              tunnel: [w159 w171] -> w143
              tunnel: w135 -> [w153 w168]
              tunnel: w128 -> [w152 w169]
              tunnel: [w151 w166] -> w134
              frame 0 {
                n39 = call "AlliGator Add Image to Accumulated Image.vi"("Image Name"="Channel 2 Accumulated Image Min", "Error In"=w156, "Dataset Index"=w150, "Accumulated Image Sum (in("=w152, "New Image"=w153) -> ("Error Out"=w154:errorcluster, "Accumulated Image Sum (out)"=w151:T5)  [unwired: 5 in]
                n40 = call "AlliGator Add Image to Accumulated Image.vi"("Image Name"="Channel 2 Accumulated Image Max", "Error In"=w156, "Dataset Index"=w150, "Accumulated Image Sum (in("=w161, "New Image"=w162) -> ("Error Out"=w160:errorcluster, "Accumulated Image Sum (out)"=w159:T5)  [unwired: 5 in]
                n41 = Merge Errors(w160, w154) -> (w155:errorcluster)
              }
              frame 1, Default {
                n42 = call "IMAQ Compare"("Operator"=T2."Min", "error in (no error)"=w167, "Image Src B"=w168, "Image Dst"=w169, "Image Src A"=w169) -> ("error out"=w164:errorcluster, "Image Dst Out"=w166:T5)  [unwired: 5 in]
                n43 = call "IMAQ Compare"("Operator"=T2."Max", "error in (no error)"=w167, "Image Src B"=w173, "Image Dst"=w170, "Image Src A"=w170) -> ("error out"=w172:errorcluster, "Image Dst Out"=w171:T5)  [unwired: 5 in]
                n44 = Merge Errors(w172, w164) -> (w165:errorcluster)
              }
            }
            n45 = for {
              tunnel: w140 -> [w185] mode=indexing
              tunnel: w139 -> [w184]
              tunnel: [w183] -> w146 mode=indexing
              tunnel: w126 -> [w182]
              tunnel: w142 -> [w181]
              tunnel: "Channel 2 Accumulated Image Array %d" ("Image Name") -> [w180]
              tunnel: [w176] -> w147 mode=indexing
              workers-P: w141 -> [_]
              tunnel: w137 -> [w175]
              i -> [w177]
              n46 = Index Array(array=w184, index=w177) -> (element=w178:T5)
              n47 = Format Into String(format string=w180, w177) -> (resulting string=w179:string)  [unwired: 2 in, 1 out]
              n48 = call "AlliGator Add Image to Accumulated Image.vi"("Weight (1)"=w175, "Image Name"=w179, "Error In"=w182, "Dataset Index"=w181, "Accumulated Image Sum (in("=w178, "New Image"=w185) -> ("Error Out"=w183:errorcluster, "Accumulated Image Sum (out)"=w176:T5)  [unwired: 4 in]
            }
            n49 = call "AlliGator Add Image to Accumulated Image.vi"("Weight (1)"=w137, "Image Name"="Channel 2 Accumulated Sum Image", "Error In"=w126, "Dataset Index"=w142, "Accumulated Image Sum (in("=w149, "New Image"=w148) -> ("Error Out"=w145:errorcluster, "Accumulated Image Sum (out)"=w136:T5)  [unwired: 4 in]
          }
          frame False {
          }
        }
      }
      n50 = in-place-cluster #2("Current Dataset"=w61, "Current Dataset Images 1.SGL Sum Image"=w75, "Accumulated Dataset Images 1.SGL Sum Image"=w76, "Current Dataset Images 1.SGL Gate Images"=w72, "Accumulated Dataset Images 1.SGL Gate Images"=w73, "Current Dataset Images 1.SGL Max Image"=w68, "Accumulated Dataset Images 1.SGL Max Image"=w65, "[Time-Series Paths]"=w47, "Dual-Channel Dataset"=w46, "Current Dataset Images 2.SGL Sum Image"=w56, "Accumulated Dataset Images 2.SGL Sum Image"=w50, "Current Dataset Images 2.SGL Gate Images"=w55, "Accumulated Dataset Images 2.SGL Gate Images"=w51, "Current Dataset Images 2.SGL Max Image"=w53, "Accumulated Dataset Images 2.SGL Max Image"=w57, "Dual-Channel Accumulated Dataset"=w46, "Current Dataset Images 1.SGL Min Image"=w43, "Accumulated Dataset Images 1.SGL Min Image"=w42, "Current Dataset Images 2.SGL Min Image"=w40, "Accumulated Dataset Images 2.SGL Min Image"=w38) -> (w36:T4)
    }
    n51 = in-place-dvr #1(w36) -> (→"AlliGator IV DVR out":refnum<data-value>, w22:errorcluster)
  }
  n52 = Merge Errors(w22, w19, w20, w2, w1, w18) -> (w17:errorcluster)
  n53 = Increment(x=w12) -> (x+1=w13:i32)
  n54 = call "Alligator Variables Storage.vi"("Get(F)/Set"=w5, "AlliGator Variable"=AlliGator_Variables_List."Number of Dataset Accumulated" ("Alligator Variable"), "Error In"=w17, "Data in"=w13) -> ("Error Out"=w11:errorcluster)  [unwired: 5 in, 2 out]
  n55 = case shown="0" w12 {
    tunnel: [w287 w290] -> w8
    tunnel: w11 -> [w285 w292]
    tunnel: w10 -> [_ w291]
    tunnel: [_ w289] -> w9
    tunnel: w5 -> [w284 _]
    frame 0 {
      # "needs to be set only once"
      n56 = call "Alligator Variables Storage.vi"("Get(F)/Set"=w284, "AlliGator Variable"=AlliGator_Variables_List."Do Averaged Datasets" ("Alligator Variable"), "Error In"=w285, "Data in"=FALSE ("Get(F)/Set")) -> ("Error Out"=w287:errorcluster)  [unwired: 5 in, 2 out]
    }
    frame 1, Default {
      n57 = call "Alligator Variables Storage.vi"("AlliGator Variable"=AlliGator_Variables_List."Array of Accumulated Dataset Paths" ("Alligator Variable"), "Error In"=w292) -> ("Error Out"=w294:errorcluster, "Data out"=w293:variant)  [unwired: 7 in, 1 out]
      n58 = Variant To Data(error in=w294, type=w291, Variant=w293) -> (data=w289:path[], error out=w290:errorcluster)
    }
  }
  n59 = case shown="False" w4 {
    tunnel: w15 -> [_ w298]
    tunnel: [w295 w297] -> w14
    tunnel: w9 -> [w295 w296]
    frame False {
    }
    frame True {
      n60 = Build Array (concatenate)(w296, w298) -> (w297:path[])
    }
  }
  n61 = call "Alligator Variables Storage.vi"("Get(F)/Set"=w5, "AlliGator Variable"=AlliGator_Variables_List."Array of Accumulated Dataset Paths" ("Alligator Variable"), "Error In"=w8, "Data in"=w14) -> ("Error Out"=→"error out":errorcluster)  [unwired: 5 in, 2 out]
